vi "SPT_List_Heuristic.vi"() -> ()   [LabVIEW 2013]
uses:
  Classes/OSSP_Problem.lvclass
  Classes/OSSP_Problem.lvclass/OSSP_Problem.ctl
  Classes/Scheduler_Class/Operation to Machine Job Tuple.vi
  Classes/Scheduler.lvclass
panel:
  in  "Problem Type":enum16{"Taillard", "Brucker", "Gueret Prins"}(ring)
  out "Makespan":u16
  out "Array 2":i32[](array[numeric])
  out "sorted array":cluster{"Numeric":u16, i32}[](array[cluster])
  out "Array":i32[](array[numeric])
  out "Processing Times":u16[][](array[numeric])
  out "output array":u16[](array[numeric])
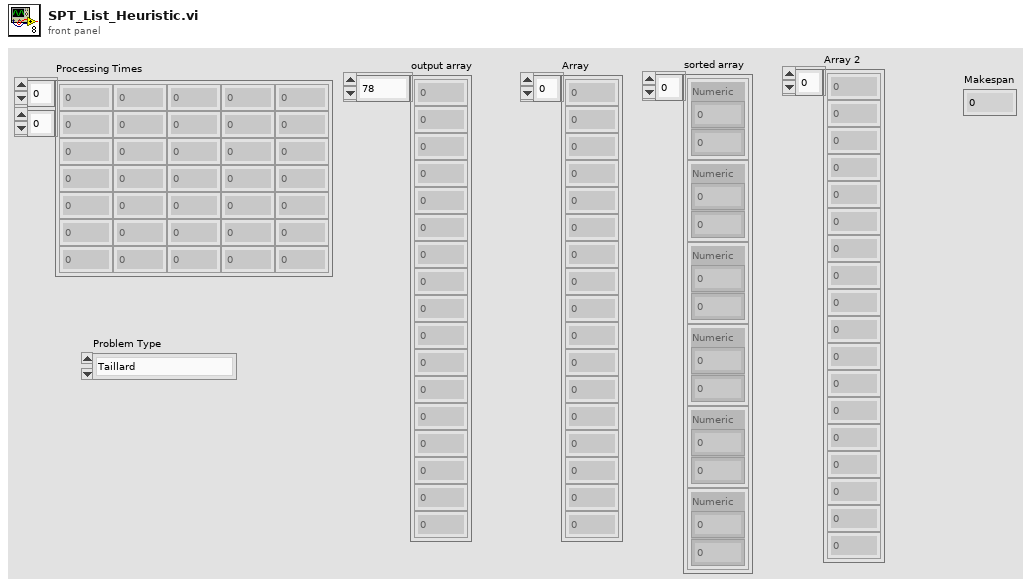
[diagram p1: front panel]
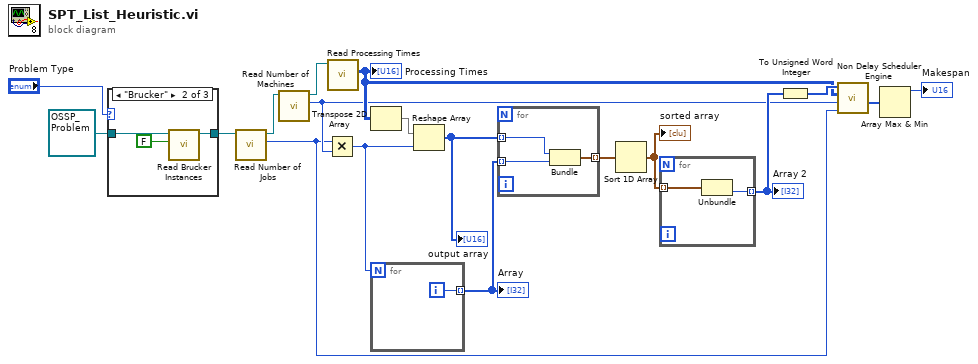
[diagram p0: block diagram]
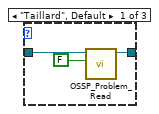
[diagram p2: hidden frame]
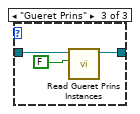
[diagram p3: hidden frame]
diagram:
  n1 = case shown="\"Brucker\"" "Problem Type" {
    tunnel: refnum<class "OSSP_Problem.lvclass"> refnum ("OSSP_Problem.lvclass In") -> [w21 w24 w27]
    tunnel: [w20 w23 w26] -> w17
    frame "Taillard", Default {
      n2 = call "OSSP_Problem_Read.vi"("Auto Mode"=FALSE, "OSSP_Problem.lvclass In"=w21) -> ("OSSP_Problem.lvclass Out"=w20:refnum<class "OSSP_Problem.lvclass">)  [unwired: 8 in, 1 out]
    }
    frame "Brucker" {
      n3 = call "Read Brucker Instances.vi"("Auto Mode"=FALSE, "OSSP_Problem in"=w24) -> ("OSSP_Problem out"=w23:refnum<class "OSSP_Problem.lvclass">)  [unwired: 8 in, 1 out]
    }
    frame "Gueret Prins" {
      n4 = call "Read Gueret Prins Instances.vi"("Auto Mode"=FALSE, "OSSP_Problem in"=w27) -> ("OSSP_Problem out"=w26:refnum<class "OSSP_Problem.lvclass">)  [unwired: 8 in, 1 out]
    }
  }
  n5 = call "Read Number of Jobs.vi"("OSSP_Problem in"=w17) -> ("Number of Jobs"=w5:i32, "OSSP_Problem out"=w16:refnum<class "OSSP_Problem.lvclass">)  [unwired: 8 in, 1 out]
  n6 = call "Read Number of Machines.vi"("OSSP_Problem in"=w16) -> ("Number of Machines"=w6:i32, "OSSP_Problem out"=w15:refnum<class "OSSP_Problem.lvclass">)  [unwired: 8 in, 1 out]
  n7 = Multiply(x=w5, y=w6) -> (x*y=w13:i32)
  n8 = call "Read Processing Times.vi"("OSSP_Problem in"=w15) -> ("Processing Times"=w7:u16[][])  [unwired: 8 in, 2 out]
  "Processing Times" <- w7
  n9 = Transpose 2D Array(2D array=w7) -> (transposed array=w14:u16[][])
  n10 = for {
    N: w13 -> [_]
    tunnel: [w28] -> w11 mode=indexing
    i -> [w28]
  }
  "Array" <- w11
  n11 = Reshape Array(w14, w13) -> (w12:u16[])
  "output array" <- w12
  n12 = for {
    tunnel: w12 -> [w31] mode=indexing
    tunnel: w11 -> [w30] mode=indexing
    tunnel: [w29] -> w10 mode=indexing
    n13 = Bundle("Numeric"=w31, w30) -> (w29:cluster{"Numeric":u16, i32})  [unwired: 1 in]
  }
  n14 = Sort 1D Array(array=w10) -> (sorted array=w1:cluster{"Numeric":u16, i32}[])
  "sorted array" <- w1
  n15 = for {
    tunnel: w1 -> [w33] mode=indexing
    tunnel: [w32] -> w9 mode=indexing
    n16 = Unbundle(w33) -> (w32:i32)  [unwired: 1 out]
  }
  "Array 2" <- w9
  n17 = To Unsigned Word Integer(number=w9) -> (unsigned 16bit integer=w8:u16[])
  n18 = call "Non Delay Scheduler Engine.vi"("Number of  Jobs"=w5, "Number of Machines"=w6, "Processing Times"=w7, "Schedule"=w8) -> ("Job Completion Times"=w4:u16[])  [unwired: 2 in, 5 out]
  n19 = Array Max & Min(array=w4) -> (max value=→"Makespan":u16)  [unwired: 3 out]
